vi "main.vi"() -> ()   [LabVIEW 2015, in "example_01.lvlib"]
uses:
  example_01.lvlib
  functional/public/_controls/event_functional.ctl
  functional/public/_controls/event_functional_command.ctl
  interfaces/dark/dark.lvclass
  interfaces/light/light.lvclass
  functional/public/interface/interface.lvclass
  functional/functional.lvlib
panel:
  out "stopped":bool
  in  "theme":enum16{"dark", "light"}(ring)=enum."light"
  in  "launch":bool
  in  "stop":bool
  out "error out":errorcluster
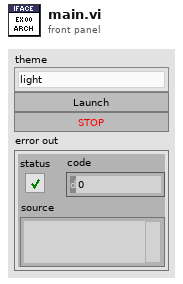
[diagram p1: front panel]
types:
  T1 = typedef "example_01.lvlib/functional.lvlib/event_functional.ctl" = cluster{"command":T2, "data":variant}
  T2 = typedef "example_01.lvlib/functional.lvlib/event_functional_command.ctl" = enum16{"<command_functional>", "--high-level", "stop", "update_hmi_references", "load_interface", "--functional", "do_it", "<null>"}
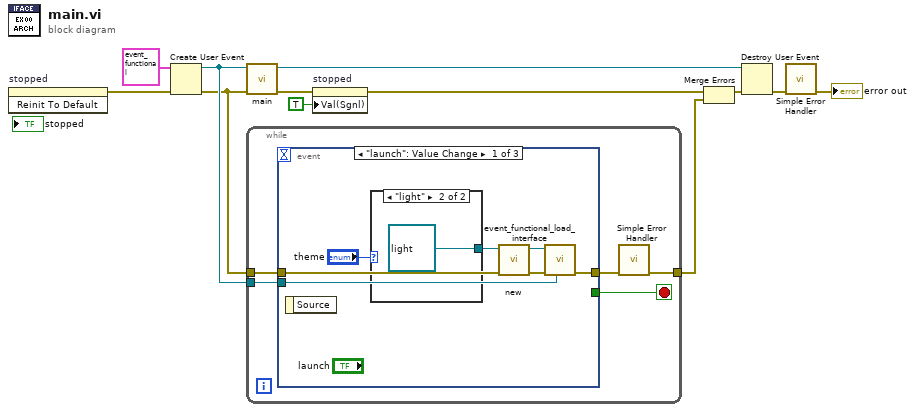
[diagram p0: block diagram]
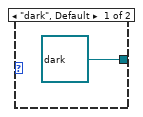
[diagram p2: hidden frame]
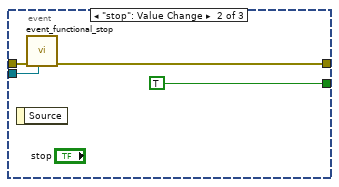
[diagram p3: hidden frame]
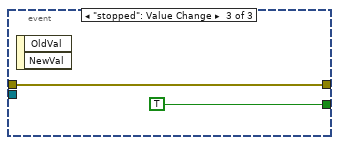
[diagram p4: hidden frame]
diagram:
  n1 = invoke on="stopped" class="Bool (strict)" method="Reinit To Default"() -> (error out=w4:errorcluster)  [unwired: 3 in, 2 out]
  n2 = Create User Event(user event datatype=T1 {"command"=enum."<command_functional>", "data"=variant} ("functional"), error in=w4) -> (user event=w6:refnum<user-event>, error out=w5:errorcluster)
  n3 = call "main.vi"("error in (no error)"=w5, "functional"=w6) -> ("error out"=w2:errorcluster)  [unwired: 9 in]
  n4 = while {
    tunnel: w5 -> [w15]
    tunnel: [w12] -> w8
    tunnel: w6 -> [w13]
    stop <- w16 stop-if-true
    n5 = event shown="[0] \"launch\": Value Change" {
      selector: _ -> [_ _ _]
      dyn-events: _ -> [_ _ _]
      timeout: _ -> [_ _ _]
      tunnel: [_ TRUE TRUE] -> w16
      tunnel: w15 -> [w20 w28 w30]
      tunnel: [w23 w27 w30] -> w14
      tunnel: w13 -> [w17 w26 _]
      event "launch": Value Change {
        n6 = event-data() -> ()  [unwired: 1 in, 1 out]
        n7 = case shown="\"light\"" "theme" {
          tunnel: [refnum<class "dark.lvclass"> refnum ("example_01.lvlib:dark.lvclass") refnum<class "light.lvclass"> refnum ("example_01.lvlib:light.lvclass")] -> w18
          frame "dark", Default {
          }
          frame "light" {
          }
        }
        n8 = call-dynamic "new.vi"("error in (no error)"=w20, "interface in"=w18) -> ("error out"=w19:errorcluster, "interface out"=w21:refnum<class "interface.lvclass">)  [unwired: 8 in]
        n9 = call "event_functional_load_interface.vi"("functional"=w17, "error in (no error)"=w19, "interface in"=w21) -> ("error out"=w23:errorcluster)  [unwired: 8 in]
      }
      event "stop": Value Change {
        n10 = event-data() -> ()  [unwired: 1 in, 1 out]
        n11 = call "event_functional_stop.vi"("functional"=w26, "error in (no error)"=w28) -> ("error out"=w27:errorcluster)  [unwired: 9 in]
      }
      event "stopped": Value Change {
        n12 = event-data() -> ()  [unwired: 1 in, 2 out]
      }
    }
    n13 = call <vilib>:"Simple Error Handler.vi"("error in (no error)"=w14) -> ("error out"=w12:errorcluster)  [unwired: 4 in, 4 out]
  }
  n14 = property on="stopped" class="Bool (strict)"(error in=w2, "Val(Sgnl)"=TRUE ("Value (Signaling)")) -> (error out=w1:errorcluster)  [unwired: 1 in, 1 out]
  n15 = Merge Errors(w1, w8) -> (w10:errorcluster)
  n16 = Destroy User Event(user event=w6, error in=w10) -> (error out=w9:errorcluster)
  n17 = call <vilib>:"Simple Error Handler.vi"("error in (no error)"=w9) -> ("error out"=→"error out":errorcluster)  [unwired: 4 in, 4 out]
